vi "Subvi FIFOOUT debug.vi"   [LabVIEW 2017]
uses:
  <vilib>/rvi/Emulation/niFpgaGetClockAttributes.vi
  <vilib>/rvi/Emulation/niFpgaSctlEmulationGetInTimedLoop.vi
  <vilib>/rvi/Emulation/niFpgaEmulationReportErrorSimple.vi
  GV preframegate.vi
  <vilib>/rvi/Emulation/niFpgaCriticalErrorInLSC.vi
  <vilib>/rvi/interface/RandomDataEmulation/niFpgaRandomDataHandleErrors.vi
  <vilib>/rvi/DataTransferAndStorage/Container/XNode/niFpgaContainer.xnode
  <vilib>/rvi/interface/RandomDataEmulation/nirviRandomDataFpgaReadWriteTemplate.vi
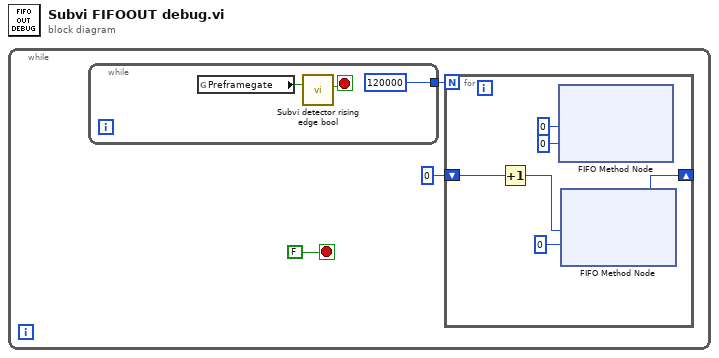
[diagram p0: block diagram]
diagram:
  n1 = while {
    stop <- FALSE stop-if-true
    n2 = while {
      tunnel: [u32 120000 ("y")] -> w1
      stop <- w4 stop-if-true
      n3 = global read "GV preframegate.vi" "Preframegate"() -> (w5:bool)
      n4 = call "Subvi detector rising edge bool.vi"("Input"=w5) -> ("Output"=w4:bool)  [unwired: 10 in]
    }
    n5 = for {
      N: w1 -> [_]
      shift-right: [w8] -> _
      shift-left: u32 0 -> [w11]
      n6 = Increment(x=w11) -> (x+1=w8:u32)
      n7 = xnode ("FIFO Method Node")("Element"=u32 0, "Timeout"=0) -> ()  [unwired: 1 in, 2 out]
      n8 = xnode ("FIFO Method Node")("Element"=w8, "Timeout"=0) -> ()  [unwired: 1 in, 2 out]
    }
  }
